vi "createTaskStack.vi"(8 "error in (no error)":errorcluster, 11 "BuildWorker in":refnum<class "BuildWorker.lvclass">) -> (0 "error out":errorcluster, 3 "BuildWorker out":refnum<class "BuildWorker.lvclass">)   [LabVIEW 2017, in "BuildWorker.lvlib" / "BuildWorker.lvclass"]
uses:
  BuildWorker.lvclass
  Classes/Task Interface/Task/Task.lvclass
  BuildWorker.lvclass/BuildWorker.ctl
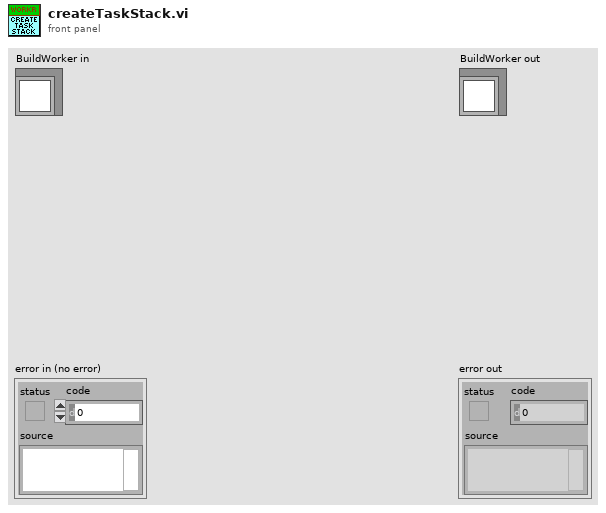
[diagram p1: front panel]
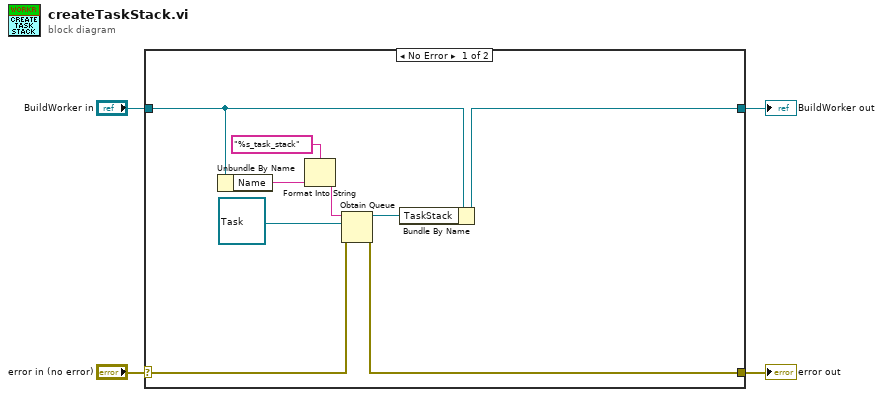
[diagram p0: block diagram]
diagram:
  n1 = case shown="No Error" "error in (no error)" {
    selector: "error in (no error)" -> [w13 w15]
    tunnel: [w12 w15] -> w3
    tunnel: [w7 w14] -> w1
    tunnel: "BuildWorker in" -> [w11 w14]
    frame No Error {
      n2 = Unbundle By Name(w11) -> ("Name"=w10:string)
      n3 = Format Into String(format string="%s_task_stack", w10) -> (resulting string=w9:string)  [unwired: 2 in, 1 out]
      n4 = Obtain Queue(name (unnamed)=w9, element data type=refnum<class "Task.lvclass"> refnum ("Task Interface.lvlib:Task.lvclass"), error in (no error)=w13) -> (queue out=w6:refnum<queue>, error out=w12:errorcluster)  [unwired: 2 in, 1 out]
      n5 = Bundle By Name(cluster=w11, "TaskStack"=w6) -> (w7:refnum<class "BuildWorker.lvclass">)
    }
    frame Error {
    }
  }
  "error out" <- w3
  "BuildWorker out" <- w1
